vi "MP-Update MultiAxis CMD.vi"(8 "Value":i32, 9 "Axis No.":u8, 10 "command name":string, 11 "CMD LUT":variant) -> (2 "Command out":string)   [LabVIEW 2026, in "MicroPulse_Driver.lvlib"]
uses:
  MicroPulse_Driver.lvlib
  <vilib>/Utility/error.llb/Trim Whitespace One-Sided.vi
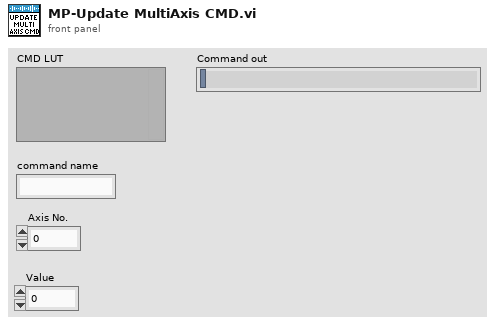
[diagram p1: front panel]
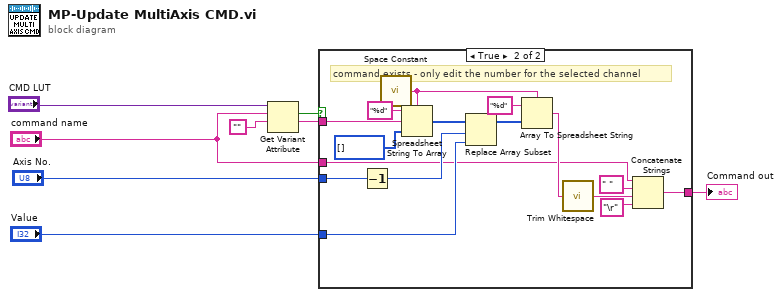
[diagram p0: block diagram]
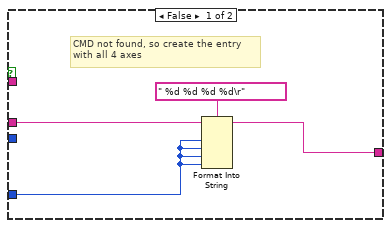
[diagram p2: hidden frame]
diagram:
  n1 = Get Variant Attribute(Variant="CMD LUT", name="command name", default value (empty Variant)="") -> (found=w5:bool, value=w6:string)  [unwired: 1 in, 2 out]
  n2 = case shown="True" w5 {
    tunnel: [w12 w18] -> w2
    tunnel: w6 -> [_ w17]
    tunnel: "Value" -> [w10 w24]
    tunnel: "Axis No." -> [_ w26]
    tunnel: "command name" -> [w9 w13]
    frame False {
      # "CMD not found, so create the entry\nwith all 4 axes"
      n3 = Format Into String(format string=" %d %d %d %d\r", initial string=w9, w10, w10, w10, w10) -> (resulting string=w12:string)  [unwired: 1 in, 1 out]
    }
    frame True {
      # "command exists - only edit the number for the selected channel"
      n4 = Decrement(x=w26) -> (x-1=w25:u8)
      n5 = call <vilib>:"Space Constant.vi"() -> ("String"=w22:string)
      n6 = Spreadsheet String To Array(delimiter (Tab)=w22, format string="%d", spreadsheet string=w17, array type (2D Dbl)=u16[] []) -> (array=w27:u16[])
      n7 = Replace Array Subset(array=w27, new element=w24, index=w25) -> (w23:u16[])
      n8 = Array To Spreadsheet String(delimiter (Tab)=w22, array=w23, 3:"%d" ("format string")) -> (spreadsheet string=w20:string)
      n9 = call <vilib>:"Trim Whitespace.vi"("string"=w20) -> ("trimmed string"=w14:string)  [unwired: 1 in]
      n10 = Concatenate Strings(w13, " " ("string"), w14, "\r" ("string")) -> (w18:string)
    }
  }
  "Command out" <- w2
